vi "FTW-Endpoint-Ask.vi"(0 "FTW Endpoint":refnum<class "FTW-Endpoint.lvclass">, 5 "Request Header":string, 7 "Request Body":string, 9 "Timeout":i32 format="%dmsec", 11 "error in":errorcluster) -> (4 "FTW Endpoint out":refnum<class "FTW-Endpoint.lvclass">, 6 "Response Header":string, 8 "Response Body":string, 10 "Timed out?":bool, 15 "error out":errorcluster)   [LabVIEW 2012, in "FTW-Actor.lvlib" / "FTW-Endpoint.lvclass"]
uses:
  FTW-Endpoint.lvclass
panel:
  # "Inputs"
  # "Outputs"
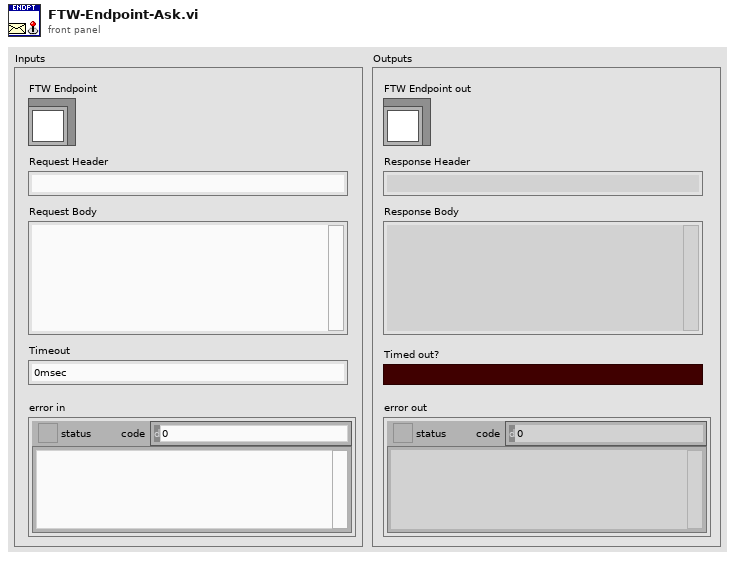
[diagram p1: front panel]
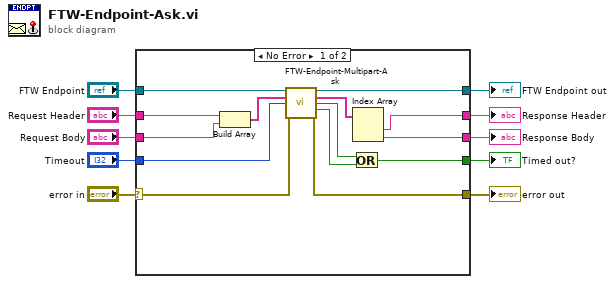
[diagram p0: block diagram]
diagram:
  n1 = case shown="No Error" "error in" {
    selector: "error in" -> [w20 w26]
    tunnel: [w19 w26] -> w10
    tunnel: [w21 w25] -> w8
    tunnel: "FTW Endpoint" -> [w22 w25]
    tunnel: [w14 _] -> w6
    tunnel: "Timeout" -> [w17 _]
    tunnel: "Request Header" -> [w24 _]
    tunnel: "Request Body" -> [w23 _]
    tunnel: [w12 _] -> w2
    tunnel: [w11 _] -> w1
    frame No Error {
      n2 = Build Array(w24, w23) -> (w18:string[])
      n3 = call-dynamic "FTW-Endpoint-Multipart-Ask.vi"("FTW Endpoint"=w22, "Multipart Message"=w18, "Read Timeout"=w17, "error in"=w20) -> ("FTW Endpoint out"=w21:refnum<class "FTW-Endpoint.lvclass">, "Reply"=w13:string[], "Read Timed out?"=w16:bool, "Write Timed out?"=w15:bool, "error out"=w19:errorcluster)  [unwired: 7 in]
      n4 = Or(x=w16, y=w15) -> (x .or. y?=w14:bool)
      n5 = Index Array(array=w13) -> (element #1=w12:string, element #2=w11:string)  [unwired: 2 in]
    }
    frame Error {
    }
  }
  "error out" <- w10
  "FTW Endpoint out" <- w8
  "Timed out?" <- w6
  "Response Header" <- w2
  "Response Body" <- w1
